vi "Finalize Settings 1.0.vi"(8 "error in (no error)":errorcluster, 11 "configuration 1.0":cluster{"processor":i32, "priority offset":i16}={"processor"=-2, "priority offset"=0}) -> (0 "error out":errorcluster, 2 "settings version":T1, 3 "settings 1.0":cluster{"key":string, "value":string}[](array[cluster]))   [LabVIEW 2019, in "DSF Core.lvlib" / "Thread Configuration.lvclass"]
uses:
  Thread Configuration.lvclass
  Typedefs/DSF Version Info.ctl
  DSF Core.lvlib
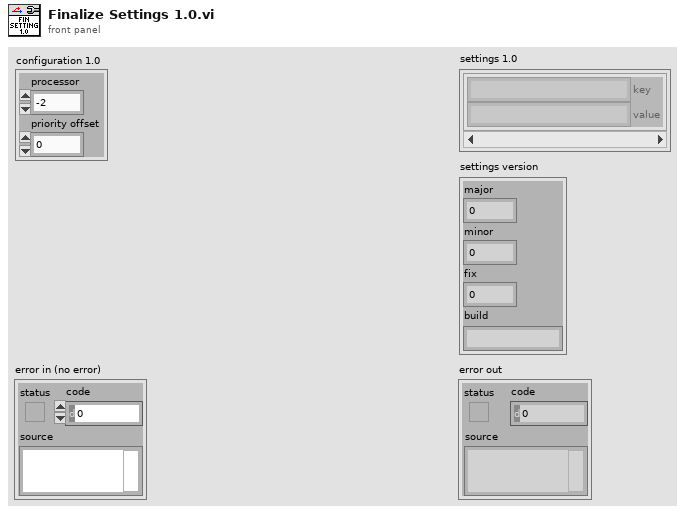
[diagram p1: front panel]
types:
  T1 = typedef "DSF Core.lvlib/DSF Version Info.ctl" = cluster{"major":u32, "minor":u32, "fix":u32, "build":string}
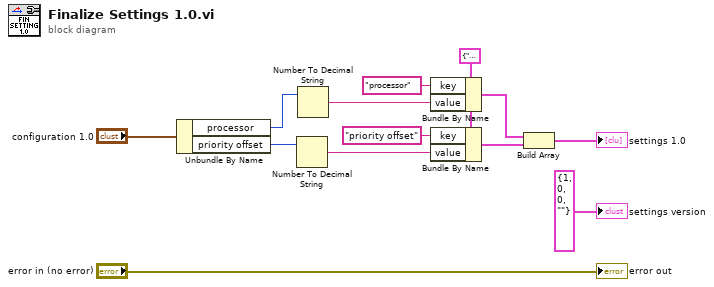
[diagram p0: block diagram]
diagram:
  w3 = cluster{"key":string, "value":string} {"key"="", "value"=""} ("setting")
  n1 = Unbundle By Name("configuration 1.0") -> ("processor"=w2:i32, "priority offset"=w8:i16)
  n2 = Number To Decimal String(number=w8) -> (decimal integer string=w9:string)  [unwired: 1 in]
  n3 = Number To Decimal String(number=w2) -> (decimal integer string=w1:string)  [unwired: 1 in]
  n4 = Bundle By Name(cluster=w3, "key"="processor", "value"=w1) -> (w13:cluster{"key":string, "value":string})
  n5 = Bundle By Name(cluster=w3, "key"="priority offset", "value"=w9) -> (w12:cluster{"key":string, "value":string})
  n6 = Build Array(w13, w12) -> (→"settings 1.0":cluster{"key":string, "value":string}[])
  "error out" <- "error in (no error)"
  "settings version" <- T1 {"major"=1, "minor"=0, "fix"=0, "build"=""} ("settings version")
